vi "Debug_Convert_Data_to_String.vi"(8 "error in (no error)":errorcluster, 11 "AB_Source_Container in":refnum<class "AB_Source_Container.lvclass">) -> (0 "error out":errorcluster, 1 "classData":string, 2 "sourceType":string, 3 "AB_Source_Container out":refnum<class "AB_Source_Container.lvclass">)   [LabVIEW 2020, in "AB_Source_Container.lvclass"]
uses:
  <vilib>/AppBuilder/AB_Classes/Source/Container/AB_Source_Container.lvclass
  <vilib>/AppBuilder/AB_Classes/Source/Container/AB_Source_Container.lvclass/AB_Source_Container.ctl
  <vilib>/AppBuilder/AB_Classes/Source/AB_Source.lvclass
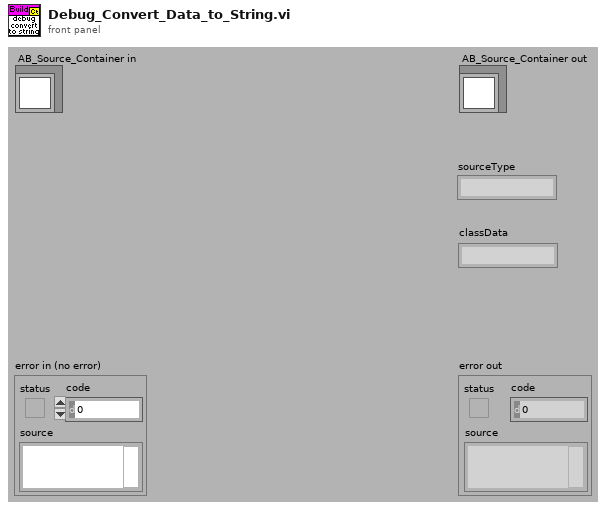
[diagram p1: front panel]
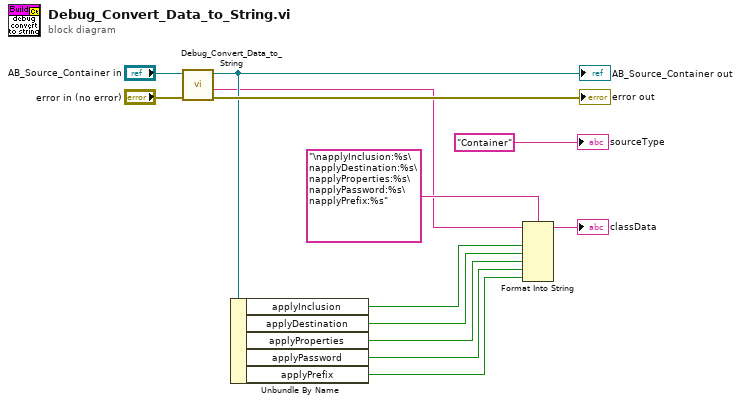
[diagram p0: block diagram]
diagram:
  n1 = call-parent "Debug_Convert_Data_to_String.vi"("error in (no error)"="error in (no error)", "AB_Source in"="AB_Source_Container in") -> ("error out"=→"error out":errorcluster, "classData"=w1:string, "AB_Source out"=w4:refnum<class "AB_Source_Container.lvclass">)  [unwired: 7 out]
  "AB_Source_Container out" <- w4
  n2 = Unbundle By Name(w4) -> ("applyInclusion"=w9:bool, "applyDestination"=w8:bool, "applyProperties"=w7:bool, "applyPassword"=w6:bool, "applyPrefix"=w5:bool)
  n3 = Format Into String(format string="\napplyInclusion:%s\napplyDestination:%s\napplyProperties:%s\napplyPassword:%s\napplyPrefix:%s", initial string=w1, w9, w8, w7, w6, w5) -> (resulting string=→"classData":string)  [unwired: 1 in, 1 out]
  "sourceType" <- "Container"
